vi "StopIfCan.vi"(11 "In Task":T1) -> (3 "Out Task":T1)   [LabVIEW 2012]
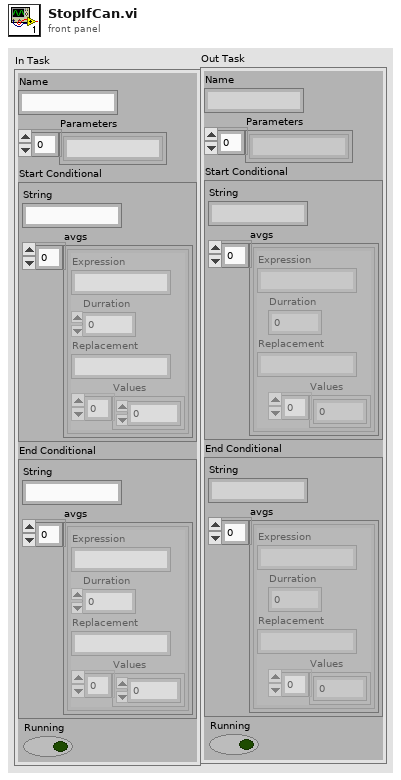
[diagram p1: front panel]
types:
  T1 = cluster{"Name":string, "Parameters":string[], "Start Conditional":cluster{"String":string, "avgs":cluster{"Expression":string, "Durration":dbl, "Replacement":string, "Values":dbl[]}[]}, "End Conditional":cluster{"String":string, "avgs":cluster{"Expression":string, "Durration":dbl, "Replacement":string, "Values":dbl[]}[]}, "Running":bool}
  T2 = cluster{"String":string, "avgs":cluster{"Expression":string, "Durration":dbl, "Replacement":string, "Values":dbl[]}[]}
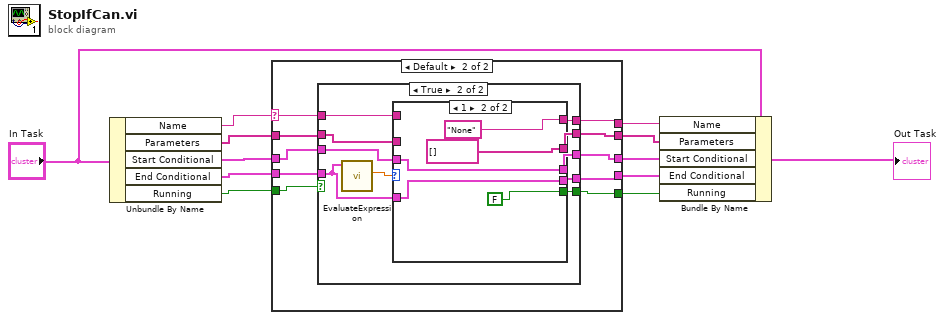
[diagram p0: block diagram]
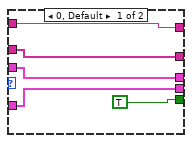
[diagram p4: hidden frame]
diagram:
  n1 = Unbundle By Name("In Task") -> ("Name"=w6:string, "Parameters"=w4:string[], "Start Conditional"=w5:T2, "End Conditional"=w3:T2, "Running"=w7:bool)
  n2 = case shown="Default" w6 {
    selector: w6 -> [w16 w19]
    tunnel: w3 -> [w13 w24]
    tunnel: w4 -> [w15 w20]
    tunnel: w5 -> [w14 w25]
    tunnel: [w17 w26] -> w12
    tunnel: w7 -> [w17 w27]
    tunnel: [w16 w18] -> w8
    tunnel: [w15 w21] -> w9
    tunnel: [w14 w22] -> w10
    tunnel: [w13 w23] -> w11
    frame "None" {
    }
    frame Default {
      n3 = case shown="True" w27 {
        selector: w27 -> [w28 _]
        tunnel: [w28 w41] -> w26
        tunnel: w25 -> [w31 w38]
        tunnel: w24 -> [w32 w36]
        tunnel: [w32 w35] -> w23
        tunnel: [w31 w37] -> w22
        tunnel: w20 -> [w30 w34]
        tunnel: [w30 w39] -> w21
        tunnel: w19 -> [w29 w33]
        tunnel: [w29 w40] -> w18
        frame False {
        }
        frame True {
          n4 = call "EvaluateExpression.vi"("Parsed Expression"=w36) -> ("Result"=w42:dbl)  [unwired: 9 in, 1 out]
          n5 = case shown="1" w42 {
            tunnel: [TRUE FALSE] -> w41
            tunnel: [w43 "None"] -> w40
            tunnel: [w44 string[] [] ("Parameters")] -> w39
            tunnel: w38 -> [w45 w49]
            tunnel: [w45 w49] -> w37
            tunnel: w36 -> [w46 w48]
            tunnel: [w46 w48] -> w35
            tunnel: w34 -> [w44 _]
            tunnel: w33 -> [w43 _]
            frame 0, Default {
            }
            frame 1 {
            }
          }
        }
      }
    }
  }
  n6 = Bundle By Name(cluster="In Task", "Name"=w8, "Parameters"=w9, "Start Conditional"=w10, "End Conditional"=w11, "Running"=w12) -> (→"Out Task":T1)
